vi "Utility Default Instrument Setup.vi"(0 "VISA resource name":refnum<visa-resource-name>, 11 "error in (no error)":errorcluster) -> (4 "VISA resource name out":refnum<visa-resource-name>, 15 "error out":errorcluster)   [LabVIEW 2011, in "Stanford Research PS300 Series.lvlib"]
doc: "This Utility VI sends a default command string to the instrument whenever a new VISA session is opened, or the instrument is reset. This VI is intended to be used as a subVI for the SRS PS3xx Initialize and SRS PS3xx Reset VI's. Altering this VI could cause these two VI's to operate incorrectly.\n\nNotes*: The factory default setups are shown below:\n Voltage Set - 0 V\n Voltage Limit - 5000 V\n Current Limit - 5.25 mA\n Current Trip - 5.25 mA\n Reset Mode - Manual\n High Voltage - Off\n GPIB Address - 14 (if applicable)"
uses:
  Stanford Research PS300 Series.lvlib
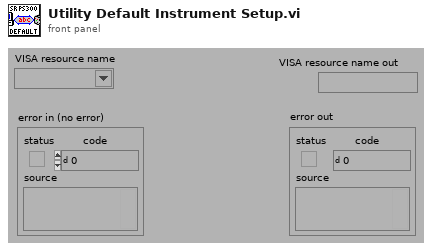
[diagram p1: front panel]
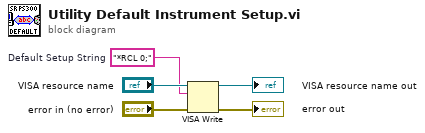
[diagram p0: block diagram]
diagram:
  w1 = "*RCL 0;"  # Default Setup String
  n1 = VISA Write(VISA resource name="VISA resource name", write buffer=w1, error in (no error)="error in (no error)") -> (VISA resource name out=→"VISA resource name out":refnum<visa-resource-name>, error out=→"error out":errorcluster)  [unwired: 1 out]
